vi "integracao_1.02.vi"() -> ()   [LabVIEW 2011]
panel:
  in  "tail n-1":dbl
  in  "tail":dbl
  out "Integral 2 anter":dbl
  out "Integral 2 n-1":dbl
  out "Area  pico":dbl
  out "tempo 3":dbl
  out "Integral 3":dbl
  out "slope neg n-1":bool
  out "tempo 2":dbl
  out "Integral 2":dbl
  out "slope pos n-1":bool
  in  "picos":dbl
  out "Boolean 4":bool
  out "appended path":path
  out "String":string
  in  "Arquivo de entrada 2":path=path "C:/works/CG3000/datalog/GC3000"
  out "Array":string[](array[string])
  out "Integral":dbl
  out "pico real":bool
  out "slope negativo":bool
  out "slope positivo":bool
  out "delta tempo menor 0,025":bool
  out "sinal menor que 1":bool
  out "signal 2":dbl
  out "Boolean 3":bool
  out "tempo":dbl
  out "Boolean 2":bool
  out "Waveform Chart 2":dynamicdata(graph)
  out "Boolean":bool
  out "slop curve":dbl
  out "Result":dbl
  out "Waveform Chart":dynamicdata(graph)
  out "signal":dbl
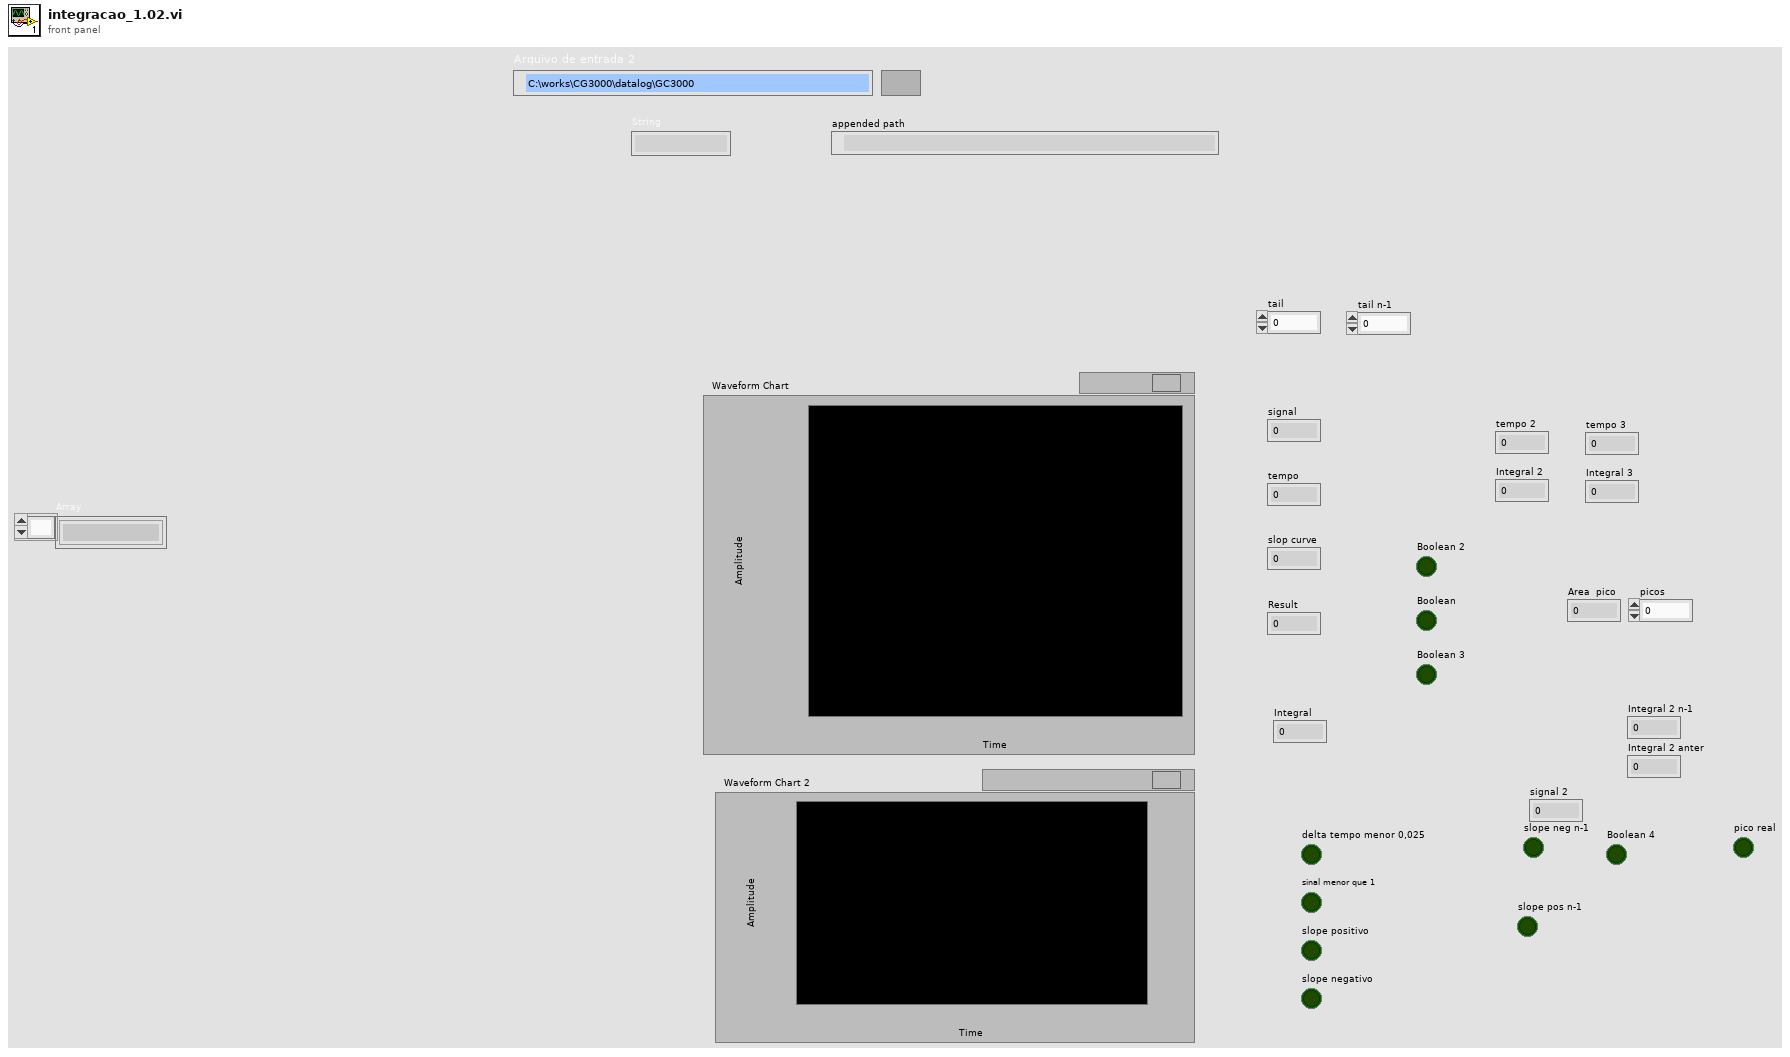
[diagram p1: front panel]
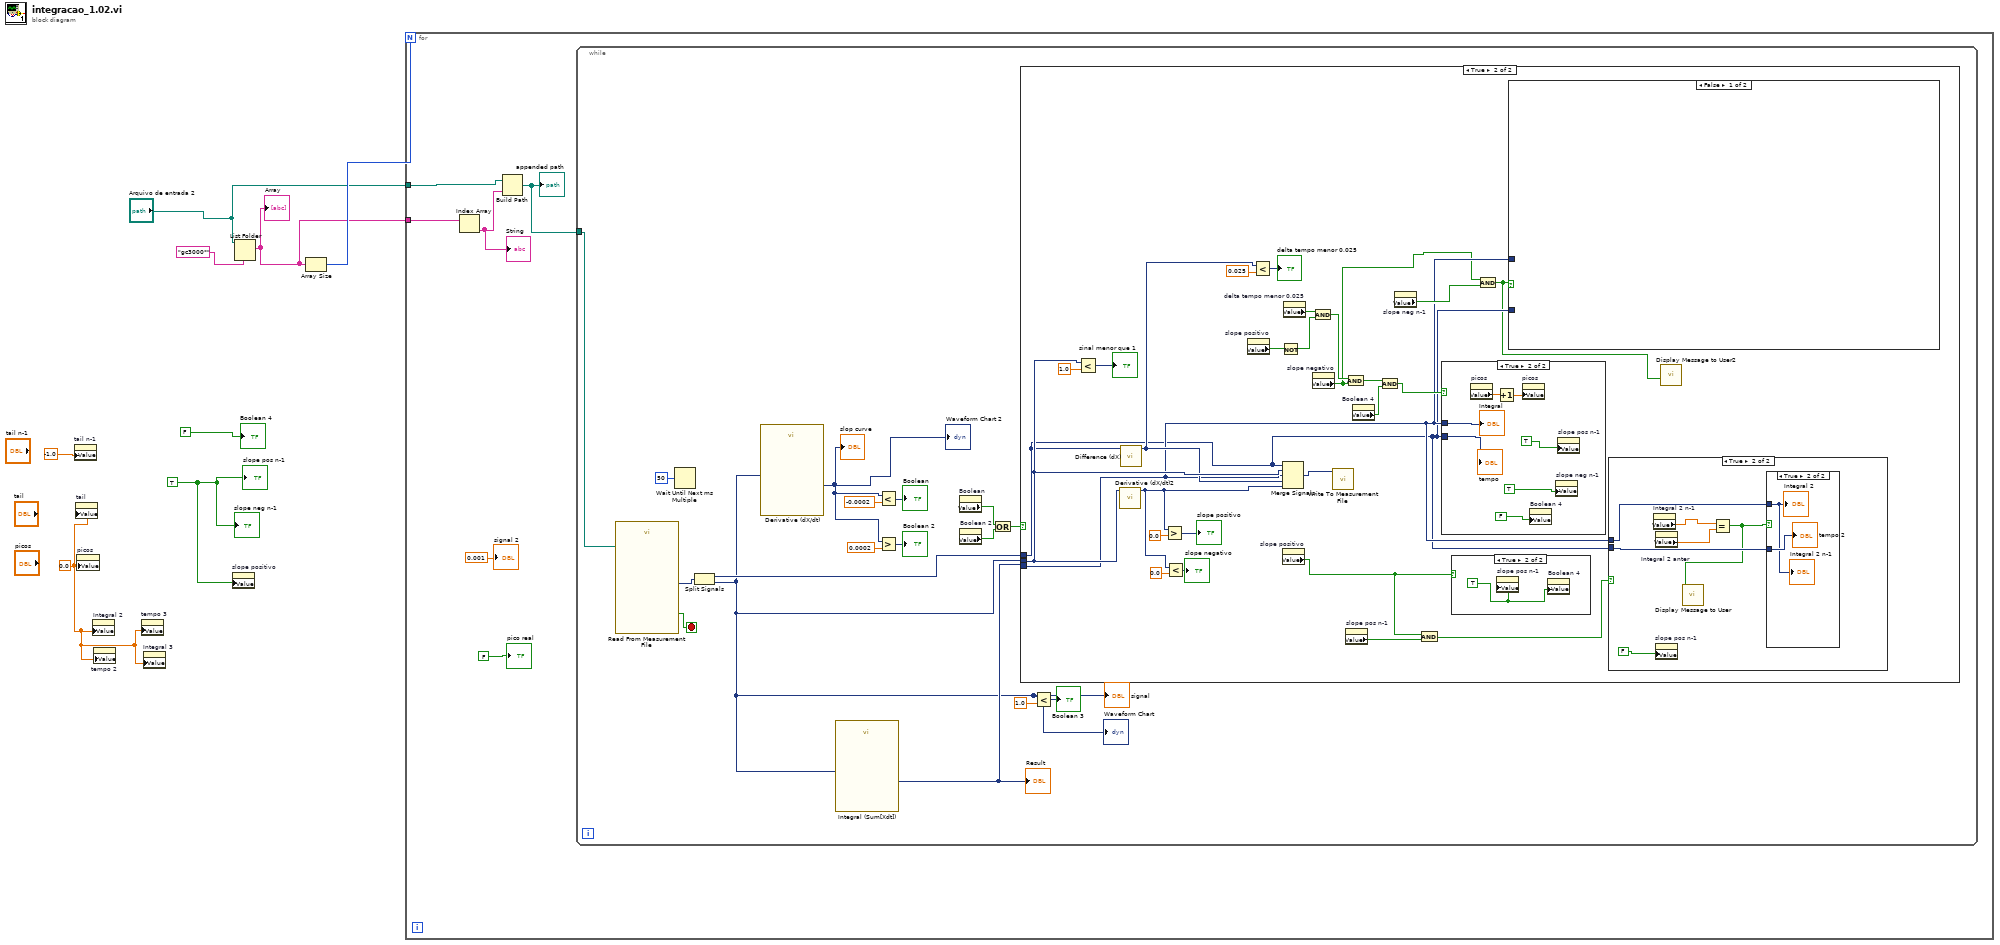
[diagram p0: block diagram]
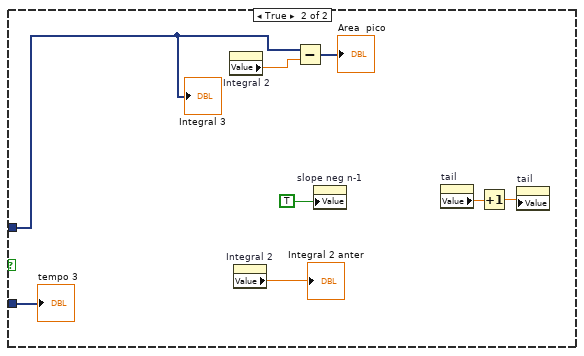
[diagram p3: hidden frame]
diagram:
  w1 = TRUE
  w2 = 0.0 ("picos")
  n1 = property on="tail n-1" class="DigNum (strict)"("Value"=-1.0 ("picos")) -> ()  [unwired: 2 in, 2 out]
  n2 = property on="tail" class="DigNum (strict)"("Value"=w2) -> ()  [unwired: 2 in, 2 out]
  n3 = property on="picos" class="DigNum (strict)"("Value"=w2) -> ()  [unwired: 2 in, 2 out]
  n4 = property on="Integral 2" class="DigNum (strict)"("Value"=w2) -> ()  [unwired: 2 in, 2 out]
  n5 = property on="tempo 2" class="DigNum (strict)"("Value"=w2) -> ()  [unwired: 2 in, 2 out]
  n6 = property on="tempo 3" class="DigNum (strict)"("Value"=w2) -> ()  [unwired: 2 in, 2 out]
  n7 = property on="Integral 3" class="DigNum (strict)"("Value"=w2) -> ()  [unwired: 2 in, 2 out]
  n8 = property on="slope positivo" class="Bool (strict)"("Value"=w1) -> ()  [unwired: 2 in, 2 out]
  n9 = List Folder(path="Arquivo de entrada 2", pattern="gc3000*") -> (filenames=w5:string[])  [unwired: 1 in, 4 out]
  "Array" <- w5
  n10 = Array Size(array=w5) -> (size(s)=w7:i32)
  n11 = for {
    N: w7 -> [_]
    tunnel: "Arquivo de entrada 2" -> [w9]
    tunnel: w5 -> [w11]
    n12 = Index Array(array=w11) -> (element=w12:string)  [unwired: 1 in]
    "String" <- w12
    n13 = Build Path(base path=w9, name or relative path=w12) -> (appended path=w10:path)
    "appended path" <- w10
    n14 = while {
      tunnel: w10 -> [w15]
      stop <- w31 stop-if-true
      n15 = call "Read From Measurement File"("Filename"=w15) -> ("Signals"=w25:dynamicdata, "EOF?"=w31:bool)  [unwired: 5 in, 4 out]
      n16 = Wait Until Next ms Multiple(millisecond multiple=u32 50) -> ()  [unwired: 1 out]
      n17 = Split Signals(w25) -> (w24:dynamicdata, w18:dynamicdata)  [unwired: 2 in]
      "signal" <- w18
      "Waveform Chart" <- w18
      n18 = call "Derivative (dX/dt)"("Signals"=w18) -> ("Result"=w16:dynamicdata)  [unwired: 5 in, 1 out]
      "slop curve" <- w16
      "Waveform Chart 2" <- w16
      n19 = call "Integral (Sum[Xdt])"("Signals"=w18) -> ("Result"=w20:dynamicdata)  [unwired: 5 in, 1 out]
      "Result" <- w20
      n20 = Less?(x=w16, y=-0.0002) -> (x < y?=→"Boolean":dynamicdata)
      n21 = Greater?(x=w16, y=0.0002) -> (0:→"Boolean 2":dynamicdata)
      n22 = property on="Boolean" class="Bool (strict)"() -> ("Value"=w23:bool)  [unwired: 2 in, 2 out]
      n23 = property on="Boolean 2" class="Bool (strict)"() -> ("Value"=w22:bool)  [unwired: 2 in, 2 out]
      n24 = Or(x=w23, y=w22) -> (x .or. y?=w21:bool)
      n25 = case shown="True" w21 {
        tunnel: w24 -> [_ w35]
        tunnel: w18 -> [_ w57]
        tunnel: w20 -> [_ w36]
        frame False {
        }
        frame True {
          n26 = Less?(x=w57, y=1.0) -> (x < y?=→"sinal menor que 1":dynamicdata)
          n27 = call "Derivative (dX/dt)2"("Signals"=w57) -> ("Result"=w49:dynamicdata)  [unwired: 5 in, 1 out]
          n28 = call "Difference (dX)"("Signals"=w35) -> ("Result"=w54:dynamicdata)  [unwired: 5 in, 1 out]
          n29 = Greater?(x=w49, y=0.0) -> (0:→"slope positivo":dynamicdata)
          n30 = Less?(x=w49, y=0.0) -> (x < y?=→"slope negativo":dynamicdata)
          n31 = property on="slope positivo" class="Bool (strict)"() -> ("Value"=w45:bool)  [unwired: 2 in, 2 out]
          n32 = Less?(x=w54, y=0.025) -> (x < y?=→"delta tempo menor 0,025":dynamicdata)
          n33 = Not(x=w45) -> (.not. x?=w44:bool)
          n34 = Merge Signals(w35, w57, w36, w54, w49) -> (w58:dynamicdata)
          n35 = property on="slope positivo" class="Bool (strict)"() -> ("Value"=w33:bool)  [unwired: 2 in, 2 out]
          n36 = property on="delta tempo menor 0,025" class="Bool (strict)"() -> ("Value"=w47:bool)  [unwired: 2 in, 2 out]
          n37 = And(x=w47, y=w44) -> (x .and. y?=w43:bool)
          n38 = property on="slope negativo" class="Bool (strict)"() -> ("Value"=w34:bool)  [unwired: 2 in, 2 out]
          n39 = call "Write To Measurement File"("Signals"=w58) -> ()  [unwired: 16 in, 3 out]
          n40 = And(x=w43, y=w34) -> (x .and. y?=w42:bool)
          n41 = property on="slope pos n-1" class="Bool (strict)"() -> ("Value"=w39:bool)  [unwired: 2 in, 2 out]
          n42 = property on="Boolean 4" class="Bool (strict)"() -> ("Value"=w40:bool)  [unwired: 2 in, 2 out]
          n43 = And(x=w42, y=w40) -> (x .and. y?=w41:bool)
          n44 = property on="slope neg n-1" class="Bool (strict)"() -> ("Value"=w37:bool)  [unwired: 2 in, 2 out]
          n45 = And(x=w33, y=w39) -> (x .and. y?=w38:bool)
          n46 = case shown="True" w41 {
            tunnel: w36 -> [_ w82]
            tunnel: w35 -> [_ w81]
            frame False {
            }
            frame True {
              n47 = property on="picos" class="DigNum (strict)"() -> ("Value"=w80:dbl)  [unwired: 2 in, 2 out]
              n48 = Increment(x=w80) -> (x+1=w79:dbl)
              n49 = property on="picos" class="DigNum (strict)"("Value"=w79) -> ()  [unwired: 2 in, 2 out]
              n50 = property on="Boolean 4" class="Bool (strict)"("Value"=FALSE) -> ()  [unwired: 2 in, 2 out]
              n51 = property on="slope neg n-1" class="Bool (strict)"("Value"=TRUE) -> ()  [unwired: 2 in, 2 out]
              n52 = property on="slope pos n-1" class="Bool (strict)"("Value"=TRUE) -> ()  [unwired: 2 in, 2 out]
              "Integral" <- w82
              "tempo" <- w81
            }
          }
          n53 = case shown="True" w33 {
            frame False {
            }
            frame True {
              w75 = TRUE
              n54 = property on="slope pos n-1" class="Bool (strict)"("Value"=w75) -> ()  [unwired: 2 in, 2 out]
              n55 = property on="Boolean 4" class="Bool (strict)"("Value"=w75) -> ()  [unwired: 2 in, 2 out]
            }
          }
          n56 = And(x=w34, y=w37) -> (x .and. y?=w32:bool)
          n57 = case shown="False" w32 {
            tunnel: w36 -> [_ w66]
            tunnel: w35 -> [_ w65]
            frame False {
            }
            frame True {
              n58 = property on="Integral 2" class="DigNum (strict)"() -> ("Value"=w63:dbl)  [unwired: 2 in, 2 out]
              n59 = property on="Integral 2" class="DigNum (strict)"() -> ("Value"=→"Integral 2 anter":dbl)  [unwired: 2 in, 2 out]
              n60 = Subtract(x=w66, y=w63) -> (x-y=→"Area  pico":dynamicdata)
              n61 = property on="slope neg n-1" class="Bool (strict)"("Value"=TRUE ("slope neg n-1")) -> ()  [unwired: 2 in, 2 out]
              n62 = property on="tail" class="DigNum (strict)"() -> ("Value"=w59:dbl)  [unwired: 2 in, 2 out]
              n63 = Increment(x=w59) -> (x+1=w60:dbl)
              n64 = property on="tail" class="DigNum (strict)"("Value"=w60) -> ()  [unwired: 2 in, 2 out]
              "Integral 3" <- w66
              "tempo 3" <- w65
            }
          }
          n65 = case shown="True" w38 {
            tunnel: w36 -> [_ w72]
            tunnel: w35 -> [_ w71]
            frame False {
            }
            frame True {
              n66 = property on="Integral 2 n-1" class="DigNum (strict)"() -> ("Value"=w69:dbl)  [unwired: 2 in, 2 out]
              n67 = property on="Integral 2 anter" class="DigNum (strict)"() -> ("Value"=w68:dbl)  [unwired: 2 in, 2 out]
              n68 = property on="slope pos n-1" class="Bool (strict)"("Value"=FALSE) -> ()  [unwired: 2 in, 2 out]
              n69 = Equal?(x=w69, y=w68) -> (x = y?=w67:bool)
              n70 = call "Display Message to User"("Enable"=w67) -> ()  [unwired: 9 in, 2 out]
              n71 = case shown="True" w67 {
                tunnel: w72 -> [_ w73]
                tunnel: w71 -> [_ w74]
                frame False {
                }
                frame True {
                  "Integral 2" <- w73
                  "tempo 2" <- w74
                  "Integral 2 n-1" <- w73
                }
              }
            }
          }
          n72 = call "Display Message to User2"("Enable"=w32) -> ()  [unwired: 9 in, 2 out]
        }
      }
      n73 = Less?(x=w18, y=1.0) -> (x < y?=→"Boolean 3":dynamicdata)
    }
    "signal 2" <- 0.001 ("signal 2")
    "pico real" <- FALSE ("pico real")
  }
  "Boolean 4" <- FALSE
  "slope pos n-1" <- w1
  "slope neg n-1" <- w1
